vi "CalculateTime.vi"(11 "Temperatura":i32) -> (3 "Tempo":i32)   [LabVIEW 2018]
doc: "Calcola il tempo di attesa per la preparazione del timer."
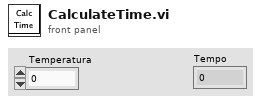
[diagram p1: front panel]
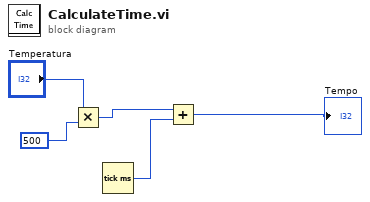
[diagram p0: block diagram]
diagram:
  n1 = Multiply(x="Temperatura", y=500) -> (x*y=w3:i32)
  n2 = Tick Count (ms)() -> (millisecond timer value=w2:u32)
  n3 = Add(x=w3, y=w2) -> (x+y=→"Tempo":u32)
